vi "VK-1701Edit Coating(in).vi"(0 "Path":string) -> ()   [LabVIEW 2009]
uses:
  <vilib>/Utility/file.llb/Read From Spreadsheet File (string).vi
panel:
  in  "Edit Coating(in) Tab":enum32{"Page 1"}(tab)
  in  "cancel":bool
  in  "ok":bool
  in  "Add Recipe":bool
  in  "Recipe List Tab":enum32{"Page 1"}(tab)
  in  "Recipe List":i32(listbox)
  in  "Path":path
  in  "Coating Name":string
  in  "delete":bool
  in  "Move up":bool
  in  "Move down":bool
  in  "Coating":i32(listbox)
  out "error out":errorcluster
  out "Path Array":string[](array[string])
  out "Recipe":string[](array[string])
  out "OKTO":bool
  # "Recipe List"
  # "Recipe File"
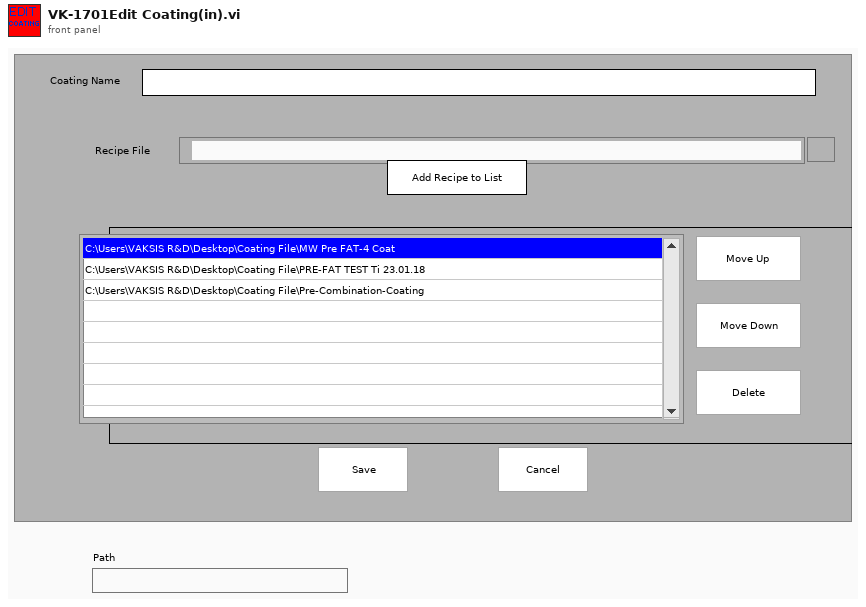
[diagram p1: front panel]
types:
  T1 = enum16{"open", "replace", "create", "open or create", "replace or create", "replace or create with confirmation"}
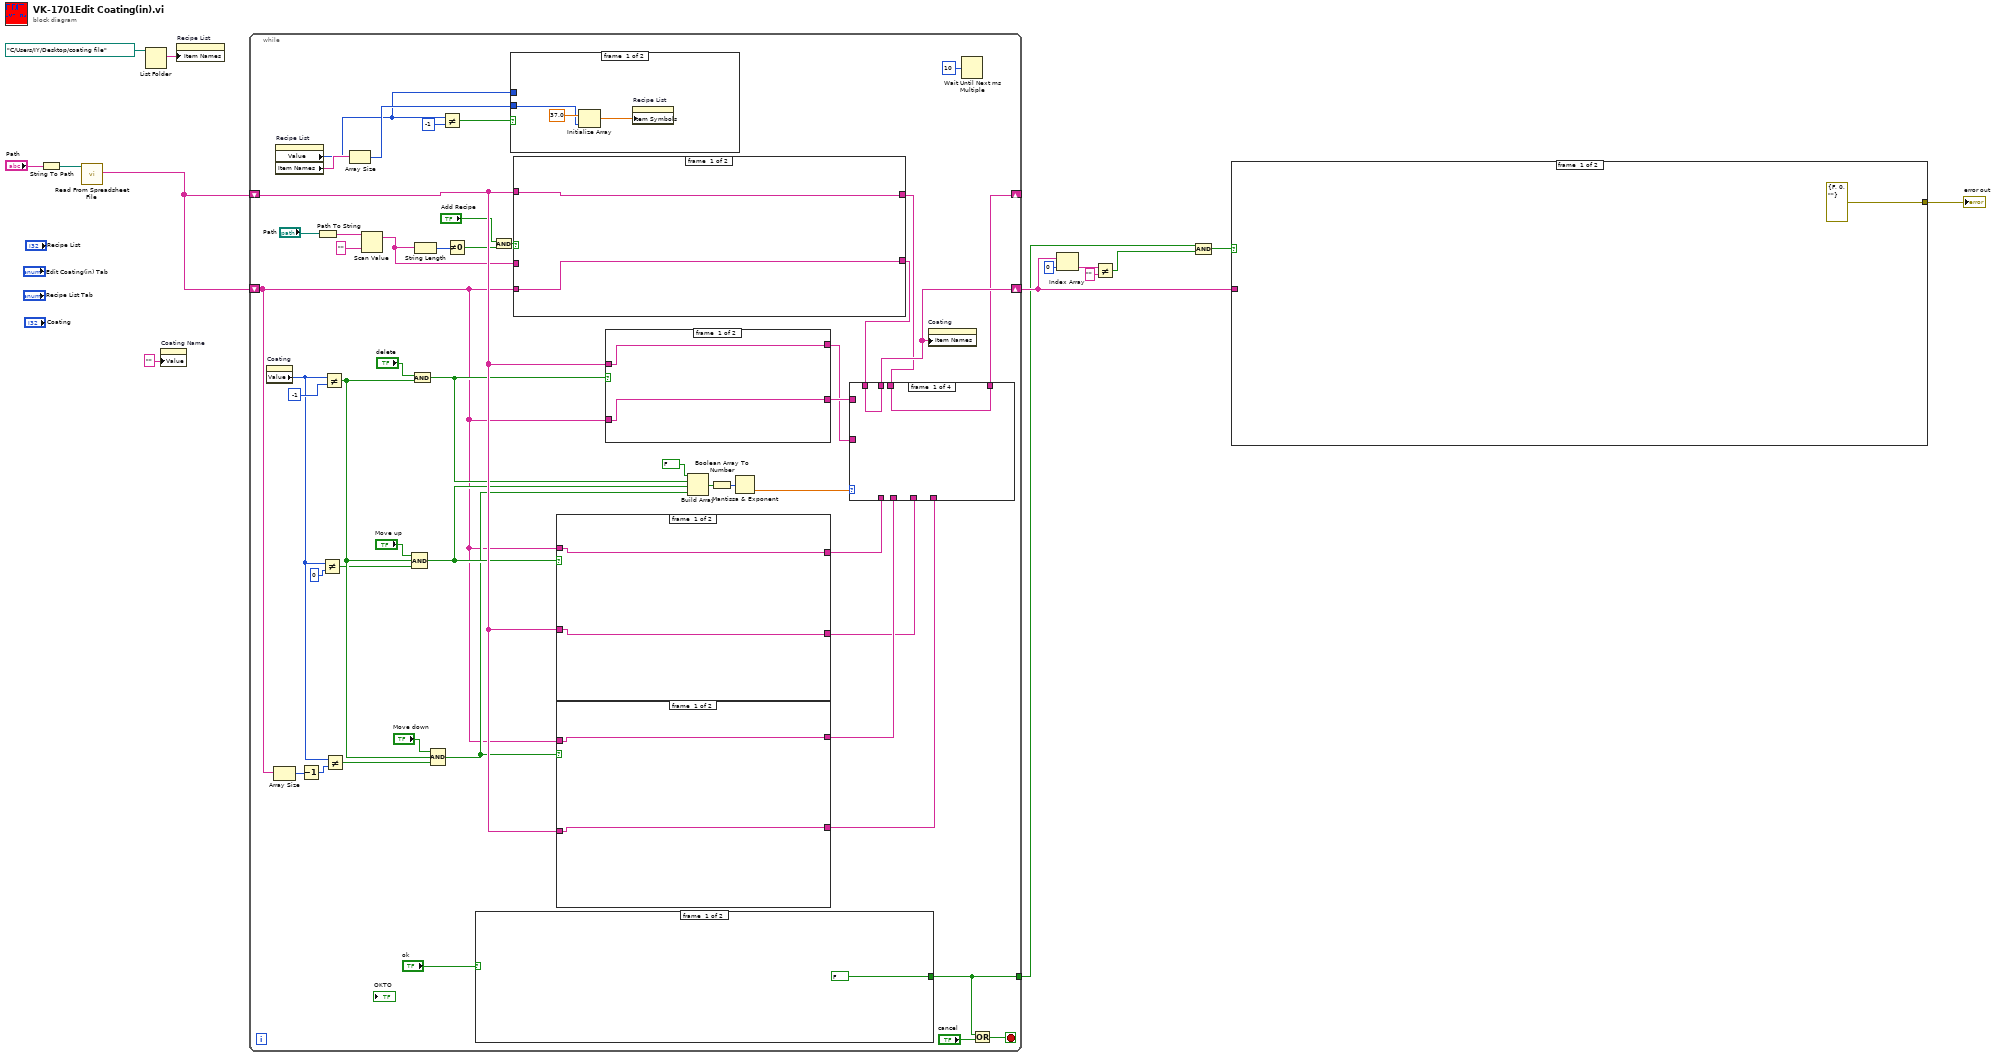
[diagram p0: block diagram]
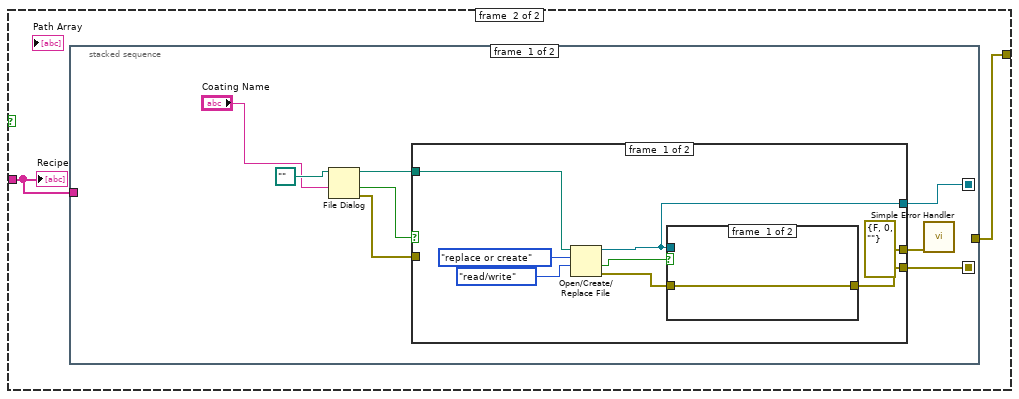
[diagram p2: hidden frame]
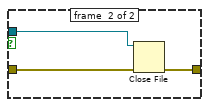
[diagram p3: hidden frame]
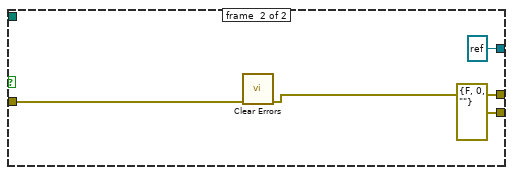
[diagram p4: hidden frame]
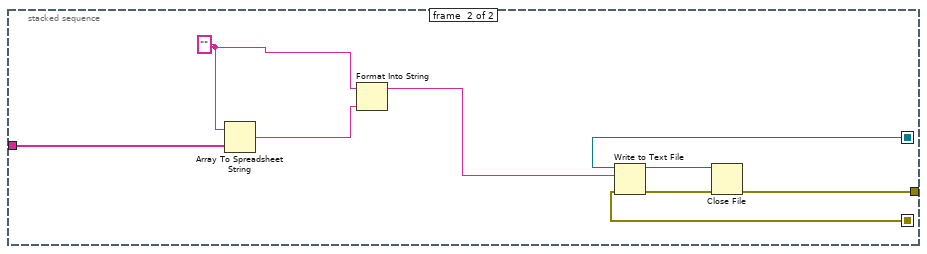
[diagram p5: hidden frame]
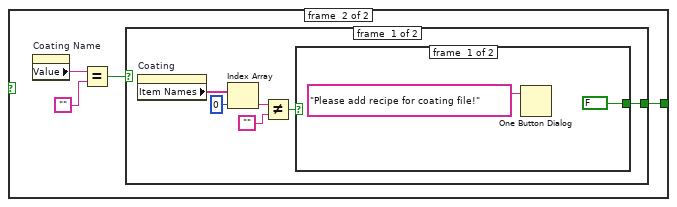
[diagram p6: hidden frame]
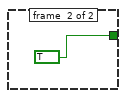
[diagram p7: hidden frame]
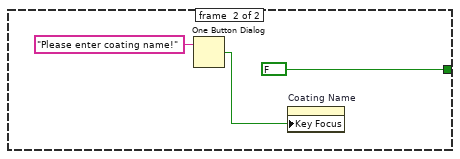
[diagram p8: hidden frame]
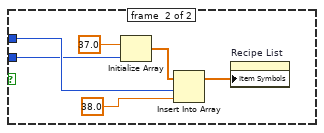
[diagram p9: hidden frame]
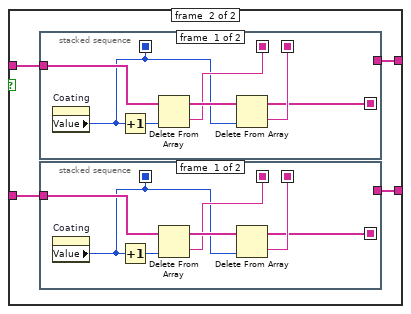
[diagram p13: hidden frame]
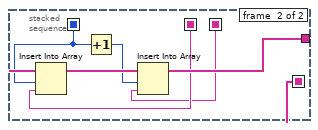
[diagram p14: hidden frame]
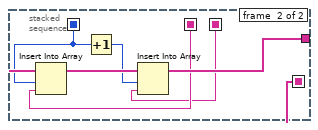
[diagram p15: hidden frame]
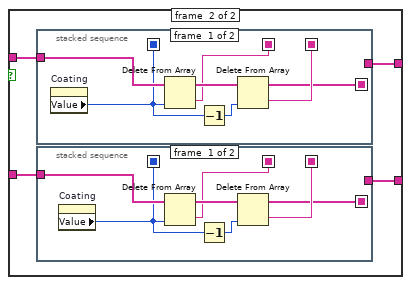
[diagram p16: hidden frame]
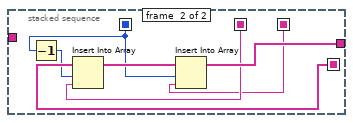
[diagram p17: hidden frame]
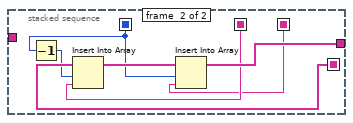
[diagram p18: hidden frame]
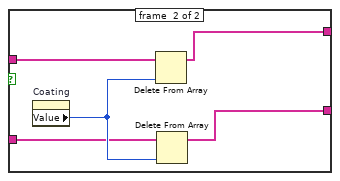
[diagram p19: hidden frame]
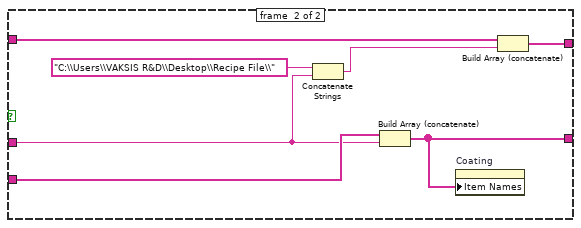
[diagram p20: hidden frame]
diagram:
  n1 = String To Path(string="Path") -> (path=w4:path)
  n2 = call-poly <vilib>:"Read From Spreadsheet File.vi"("file path (dialog if empty)"=w4) -> ("first row"=w2:string[])  [unwired: 6 in, 4 out]
  n3 = List Folder(path=path "C:/Users/IY/Desktop/coating file") -> (filenames=w7:string[])  [unwired: 3 in, 3 out]
  n4 = property on="Coating Name" class="Str"("Value"="" ("Coating Name :")) -> ()  [unwired: 2 in, 2 out]
  n5 = property on="Recipe List" class="LstBox (strict)"("Item Names"=w7) -> ()  [unwired: 2 in, 2 out]
  n6 = while {
    shift-right: [w49] -> _
    shift-left: w2 -> [w52]
    shift-right: [w53] -> w14
    shift-left: w2 -> [w33]
    tunnel: [w22] -> w5
    stop <- w61 stop-if-true
    n7 = property on="Coating" class="LstBox (strict)"() -> ("Value"=w34:i32)  [unwired: 2 in, 2 out]
    n8 = Array Size(array=w33) -> (size(s)=w32:i32)
    n9 = property on="Recipe List" class="LstBox (strict)"() -> ("Value"=w24:i32, "Item Names"=w29:string[])  [unwired: 2 in, 2 out]
    n10 = Decrement(x=w32) -> (x-1=w31:i32)
    n11 = Path To String(path="Path") -> (string=w19:string)
    n12 = Not Equal?(x=w34, y=0) -> (x != y?=w36:bool)
    n13 = Not Equal?(x=w34, y=-1) -> (x != y?=w40:bool)
    n14 = Not Equal?(x=w34, y=w31) -> (x != y?=w35:bool)
    n15 = Array Size(array=w29) -> (size(s)=w27:i32)
    n16 = Scan Value(string=w19, format string="") -> (output string=w15:string)  [unwired: 1 in, 1 out]
    n17 = And(x="delete", y=w40) -> (x .and. y?=w43:bool)
    n18 = Compound Arithmetic op=AND("Move up", w40, w36) -> (w41:bool)
    n19 = String Length(string=w15) -> (length=w17:i32)
    n20 = Compound Arithmetic op=AND("Move down", w40, w35) -> (w38:bool)
    n21 = Not Equal?(x=w24, y=-1) -> (x != y?=w28:bool)
    n22 = Not Equal To 0?(x=w17) -> (x != 0?=w16:bool)
    n23 = case shown="True" "ok" {
      tunnel: [FALSE w64] -> w22
      frame #0 {
      }
      frame #1 {
        n24 = property on="Coating Name" class="Str"() -> ("Value"=w66:string)  [unwired: 2 in, 2 out]
        n25 = Equal?(x=w66, y="") -> (x = y?=w65:bool)
        n26 = case shown="False" w65 {
          tunnel: [w68 FALSE] -> w64
          frame #0 {
            n27 = property on="Coating" class="LstBox (strict)"() -> ("Item Names"=w71:string[])  [unwired: 2 in, 2 out]
            n28 = Index Array(array=w71, index=0) -> (element=w73:string)
            n29 = Not Equal?(x=w73, y="") -> (x != y?=w69:bool)
            n30 = case shown="False" w69 {
              tunnel: [FALSE TRUE] -> w68
              frame #0 {
                n31 = One Button Dialog(message="Please add recipe for coating file!") -> ()  [unwired: 1 in, 1 out]
              }
              frame #1 {
              }
            }
          }
          frame #1 {
            n32 = One Button Dialog(message="Please enter coating name!") -> (true=w77:bool)  [unwired: 1 in]
            n33 = property on="Coating Name" class="Str"("Key Focus"=w77) -> ()  [unwired: 2 in, 2 out]
          }
        }
      }
    }
    n34 = And(x="Add Recipe", y=w16) -> (x .and. y?=w26:bool)
    n35 = case shown="False" w28 {
      tunnel: w24 -> [_ w85]
      tunnel: w27 -> [w81 w84]
      frame #0 {
        n36 = Initialize Array(37.0 ("element"), w81) -> (w80:dbl[])
        n37 = property on="Recipe List" class="LstBox (strict)"("Item Symbols"=w80) -> ()  [unwired: 2 in, 2 out]
      }
      frame #1 {
        n38 = Initialize Array(37.0 ("element"), w84) -> (w88:dbl[])
        n39 = Insert Into Array(array=w88, index=w85, new element=38.0 ("element")) -> (w83:dbl[])
        n40 = property on="Recipe List" class="LstBox (strict)"("Item Symbols"=w83) -> ()  [unwired: 2 in, 2 out]
      }
    }
    n41 = case shown="True" w26 {
      tunnel: [w173 w178] -> w50
      tunnel: [w172 w177] -> w51
      tunnel: w33 -> [w172 w180]
      tunnel: w52 -> [w173 w179]
      tunnel: w15 -> [_ w174]
      frame #0 {
      }
      frame #1 {
        n42 = Concatenate Strings("C:\\Users\\VAKSIS R&D\\Desktop\\Recipe File\\" ("string"), w174) -> (w175:string)
        n43 = Build Array (concatenate)(w180, w174) -> (w177:string[])
        n44 = property on="Coating" class="LstBox (strict)"("Item Names"=w177) -> ()  [unwired: 2 in, 2 out]
        n45 = Build Array (concatenate)(w179, w175) -> (w178:string[])
      }
    }
    n46 = case shown="True" w41 {
      tunnel: w33 -> [w132 w136]
      tunnel: [w132 w135] -> w55
      tunnel: w52 -> [w131 w134]
      tunnel: [w131 w133] -> w48
      frame #0 {
      }
      frame #1 {
        n47 = stacked-sequence {
          seq-local: [w154 _] -> [_ w159]
          seq-local: [w153 _] -> [_ w158]
          seq-local: [w152 _] -> [_ w164]
          seq-local: [w151 _] -> [_ w161]
          tunnel: w136 -> [w157 _]
          tunnel: [_ w162] -> w135
          frame #0 {
            n48 = property on="Coating" class="LstBox (strict)"() -> ("Value"=w151:i32)  [unwired: 2 in, 2 out]
            n49 = Delete From Array(array=w157, index=w151) -> (deleted portion=w154:string, array with subset deleted=w156:string[])  [unwired: 1 in]
            n50 = Decrement(x=w151) -> (x-1=w155:i32)
            n51 = Delete From Array(array=w156, index=w155) -> (deleted portion=w153:string, array with subset deleted=w152:string[])  [unwired: 1 in]
          }
          frame #1 {
            n52 = Decrement(x=w161) -> (x-1=w160:i32)
            n53 = Insert Into Array(array=w164, index=w160, new element=w159) -> (w163:string[])
            n54 = Insert Into Array(array=w163, index=w161, new element=w158) -> (w162:string[])
          }
        }
        n55 = stacked-sequence {
          seq-local: [w140 _] -> [_ w145]
          seq-local: [w139 _] -> [_ w144]
          seq-local: [w138 _] -> [_ w150]
          seq-local: [w137 _] -> [_ w147]
          tunnel: w134 -> [w143 _]
          tunnel: [_ w148] -> w133
          frame #0 {
            n56 = property on="Coating" class="LstBox (strict)"() -> ("Value"=w137:i32)  [unwired: 2 in, 2 out]
            n57 = Delete From Array(array=w143, index=w137) -> (deleted portion=w140:string, array with subset deleted=w142:string[])  [unwired: 1 in]
            n58 = Decrement(x=w137) -> (x-1=w141:i32)
            n59 = Delete From Array(array=w142, index=w141) -> (deleted portion=w139:string, array with subset deleted=w138:string[])  [unwired: 1 in]
          }
          frame #1 {
            n60 = Decrement(x=w147) -> (x-1=w146:i32)
            n61 = Insert Into Array(array=w150, index=w146, new element=w145) -> (w149:string[])
            n62 = Insert Into Array(array=w149, index=w147, new element=w144) -> (w148:string[])
          }
        }
      }
    }
    n63 = case shown="True" w38 {
      tunnel: w33 -> [w98 w102]
      tunnel: [w98 w101] -> w54
      tunnel: w52 -> [w97 w100]
      tunnel: [w97 w99] -> w46
      frame #0 {
      }
      frame #1 {
        n64 = stacked-sequence {
          seq-local: [w119 _] -> [_ w127]
          seq-local: [w121 _] -> [_ w126]
          seq-local: [w120 _] -> [_ w130]
          seq-local: [w117 _] -> [_ w124]
          tunnel: w102 -> [w122 _]
          tunnel: [_ w129] -> w101
          frame #0 {
            n65 = property on="Coating" class="LstBox (strict)"() -> ("Value"=w117:i32)  [unwired: 2 in, 2 out]
            n66 = Increment(x=w117) -> (x+1=w118:i32)
            n67 = Delete From Array(array=w122, index=w118) -> (deleted portion=w119:string, array with subset deleted=w123:string[])  [unwired: 1 in]
            n68 = Delete From Array(array=w123, index=w117) -> (deleted portion=w121:string, array with subset deleted=w120:string[])  [unwired: 1 in]
          }
          frame #1 {
            n69 = Insert Into Array(array=w130, index=w124, new element=w127) -> (w128:string[])
            n70 = Increment(x=w124) -> (x+1=w125:i32)
            n71 = Insert Into Array(array=w128, index=w125, new element=w126) -> (w129:string[])
          }
        }
        n72 = stacked-sequence {
          seq-local: [w105 _] -> [_ w113]
          seq-local: [w107 _] -> [_ w112]
          seq-local: [w106 _] -> [_ w116]
          seq-local: [w103 _] -> [_ w110]
          tunnel: w100 -> [w108 _]
          tunnel: [_ w115] -> w99
          frame #0 {
            n73 = property on="Coating" class="LstBox (strict)"() -> ("Value"=w103:i32)  [unwired: 2 in, 2 out]
            n74 = Increment(x=w103) -> (x+1=w104:i32)
            n75 = Delete From Array(array=w108, index=w104) -> (deleted portion=w105:string, array with subset deleted=w109:string[])  [unwired: 1 in]
            n76 = Delete From Array(array=w109, index=w103) -> (deleted portion=w107:string, array with subset deleted=w106:string[])  [unwired: 1 in]
          }
          frame #1 {
            n77 = Insert Into Array(array=w116, index=w110, new element=w113) -> (w114:string[])
            n78 = Increment(x=w110) -> (x+1=w111:i32)
            n79 = Insert Into Array(array=w114, index=w111, new element=w112) -> (w115:string[])
          }
        }
      }
    }
    n80 = case shown="True" w43 {
      tunnel: w52 -> [w165 w171]
      tunnel: w33 -> [w166 w169]
      tunnel: [w166 w168] -> w56
      tunnel: [w165 w167] -> w47
      frame #0 {
      }
      frame #1 {
        n81 = property on="Coating" class="LstBox (strict)"() -> ("Value"=w170:i32)  [unwired: 2 in, 2 out]
        n82 = Delete From Array(array=w171, index=w170) -> (array with subset deleted=w167:string[])  [unwired: 1 in, 1 out]
        n83 = Delete From Array(array=w169, index=w170) -> (array with subset deleted=w168:string[])  [unwired: 1 in, 1 out]
      }
    }
    n84 = Build Array(FALSE, w43, w41, w38) -> (w58:bool[])
    n85 = Boolean Array To Number(Boolean array=w58) -> (number=w59:u32)
    n86 = Mantissa & Exponent(0:w59) -> (2:w57:dbl)  [unwired: 1 out]
    n87 = case shown="0, Default" w57 {
      tunnel: w56 -> [_ w92 _ _]
      tunnel: [w90 w92 w94 w96] -> w53
      tunnel: w55 -> [_ _ w94 _]
      tunnel: w54 -> [_ _ _ w96]
      tunnel: w51 -> [w90 _ _ _]
      tunnel: w50 -> [w89 _ _ _]
      tunnel: [w89 w91 w93 w95] -> w49
      tunnel: w48 -> [_ _ w93 _]
      tunnel: w47 -> [_ w91 _ _]
      tunnel: w46 -> [_ _ _ w95]
      frame #0 {
      }
      frame #1 {
      }
      frame #2 {
      }
      frame #3 {
      }
    }
    n88 = property on="Coating" class="LstBox (strict)"("Item Names"=w53) -> ()  [unwired: 2 in, 2 out]
    n89 = Wait Until Next ms Multiple(millisecond multiple=u32 10) -> ()  [unwired: 1 out]
    n90 = Or(x=w22, y="cancel") -> (x .or. y?=w61:bool)
  }
  n91 = Index Array(array=w14, index=0) -> (element=w12:string)
  n92 = Not Equal?(x=w12, y="") -> (x != y?=w10:bool)
  n93 = Compound Arithmetic op=AND(w5, w10) -> (w9:bool)
  n94 = case shown="True" w9 {
    tunnel: w14 -> [_ w183]
    tunnel: [errorcluster {"status"=FALSE, "code"=0, "source"=""} ("error out") w182] -> w8
    frame #0 {
    }
    frame #1 {
      n95 = stacked-sequence {
        seq-local: [w191 _] -> [_ w212]
        seq-local: [w190 _] -> [_ w210]
        tunnel: w183 -> [_ w216]
        tunnel: [_ w209] -> w182
        frame #0 {
          n96 = File Dialog(9:"Coating Name", 11:path "" ("base path")) -> (0:w185:errorcluster, 1:w186:bool, 3:w189:path)  [unwired: 2 in, 4 out]
          n97 = case shown="False" w186 {
            tunnel: [w196 refnum<file> refnum ("refnum out")] -> w191
            tunnel: [w195 errorcluster {"status"=FALSE, "code"=0, "source"=""} ("error out")] -> w190
            tunnel: w189 -> [w194 _]
            tunnel: w185 -> [_ w207]
            tunnel: [errorcluster {"status"=FALSE, "code"=0, "source"=""} ("error out") w206] -> w184
            frame #0 {
              n98 = Open/Create/Replace File(file path (use dialog)=w194, operation (0:open)=T1."replace or create", access (0:read/write)=enum16{"read/write", "read-only", "write-only"}."read/write") -> (refnum out=w196:refnum<file>, cancelled=w193:bool, error out=w199:errorcluster)  [unwired: 3 in]
              n99 = case shown="True" w193 {
                tunnel: w196 -> [_ w203]
                tunnel: w199 -> [w200 w202]
                tunnel: [w200 w201] -> w195
                frame #0 {
                }
                frame #1 {
                  n100 = Close File(refnum=w203, error in=w202) -> (error out=w201:errorcluster)  [unwired: 1 out]
                }
              }
            }
            frame #1 {
              n101 = call <vilib>:"Clear Errors.vi"("error in (no error)"=w207) -> ("error out"=w206:errorcluster)  [unwired: 6 in]
            }
          }
          n102 = call <vilib>:"Simple Error Handler.vi"("error in (no error)"=w184) -> ()  [unwired: 4 in, 5 out]
        }
        frame #1 {
          w208 = "" ("format string")
          n103 = Array To Spreadsheet String(array=w216, 3:w208) -> (spreadsheet string=w215:string)  [unwired: 1 in]
          n104 = Format Into String(initial string=w208, w215) -> (resulting string=w213:string)  [unwired: 2 in, 1 out]
          n105 = Write to Text File(file (use dialog)=w212, text=w213, error in=w210) -> (refnum out=w211:refnum<file>, error out=w214:errorcluster)  [unwired: 1 in, 1 out]
          n106 = Close File(refnum=w211, error in=w214) -> (error out=w209:errorcluster)  [unwired: 1 out]
        }
      }
      "Recipe" <- w183
    }
  }
  "error out" <- w8
